vi "input safety.vi"(10 "Desired Rate":dbl, 11 "Encoder Rate":dbl) -> (2 "Safe Rate":dbl, 3 "Encoder Rate Out":dbl, 4 "Input Out of Range":bool)   [LabVIEW 2014]
panel:
  # "Make Sure a Valid Rate Is Requested"
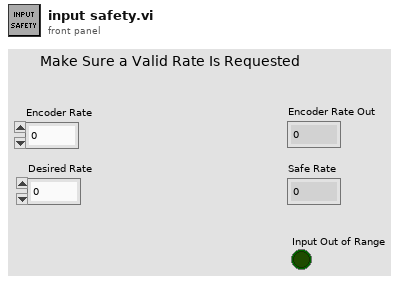
[diagram p1: front panel]
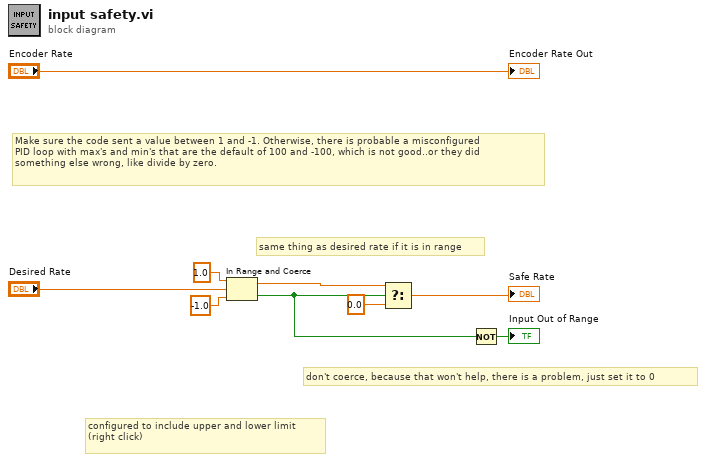
[diagram p0: block diagram]
diagram:
  # "configured to include upper and lower limit\n(right click)"
  # "same thing as desired rate if it is in range"
  # "don't coerce, because that won't help, there is a problem, just set it to 0"
  # "Make sure the code sent a value between 1 and -1. Otherwise, there is probable a misconfigured\nPID loop with max's and min's that are the default of 100 and -100, which is not good..or they did \nsomething else wrong, like divide by zero."
  n1 = In Range and Coerce(upper limit=1.0, x="Desired Rate", lower limit=-1.0 ("upper limit")) -> (coerced(x)=w5:dbl, In Range?=w2:bool)
  n2 = Select(t=w5, s=w2, f=0.0) -> (s? t:f=→"Safe Rate":dbl)
  n3 = Not(x=w2) -> (.not. x?=→"Input Out of Range":bool)
  "Encoder Rate Out" <- "Encoder Rate"
